vi "ble_read_write_characteristics.vi"() -> ()   [LabVIEW 2013]
uses:
  type_def/connection_status_bundle.ctl
  type_def/address_type.ctl
  ble_functions/ble_write_by_service_characteristic_uint8array.vi
panel:
  out "Connected":bool
  out "Device Name":string
  in  "Address Type":T1=1 items=["Public", "Random"]
  out "Handle table":string[][](array[string])
  out "Connection Status":T2={"MAC Address"="", "cnx handle"=0, "cnx flags"=0, "Address Type"=125, "Connection Interval (ms)"=125, "Timeout(ms)"=125, "Latency"=0, "bonding handle"=0} {"Address Type" items=["Public", "Random"]}
  out "Scanning":bool
  in  "Continue":bool
  in  "MAC Address":string
  in  "COM Bluegiga in":refnum<visa-resource-name>="COM13"
  out "Devices":string[][](array[string])
  out "BLED112 Dongle Info":string
  # "This VI an example of scanning for BLE devices using the \nBLED112 Bluetooth Smart Dongle by Bluegiga\nhttps://www.bluegiga.com/en-US/products/bled112-bluetooth-smart-dongle/\n\nand\nBLE (Bluetooth Low Energy) toolkit for LabVIEW\nww.\n\nInstructions:\nBefore running the VI\n1. Select the COM port for the BLED112 USB receiver\n(You can verify this in the Device Manager)\n\n2. Run the VI\n\n3. The VI will reset the dongle and scan for available BLE devices\n \n4. Introduce the MAC Address and Address Type of the device you want to connect and click in the CONTINUE button to connect with it\n\n5. The VI will read the Characteristic 0x2A00 of the Service 0x1800 which contains \nthe Device Name\n\nhttps://www.bluetooth.com/specifications/gatt/viewer?attributeXmlFile=org.bluetooth.service.generic_access.xml&u=org.bluetooth.service.generic_access.xml"
  # "SCAN"
  # "RSSI (power)"
  # "Advertising Package Type"
  # "MAC Address"
  # "Address Type"
  # "Friendly name"
  # "DEVICES FOUND"
  # "Introduce the MAC Address and Address Type of the device you want to connect and click in the CONTINUE button"
  # "CONNECT"
  # "READING DEVICE NAME"
  # "Service 0x1800\nCharacteristic 0x2A00\nDevice Name"
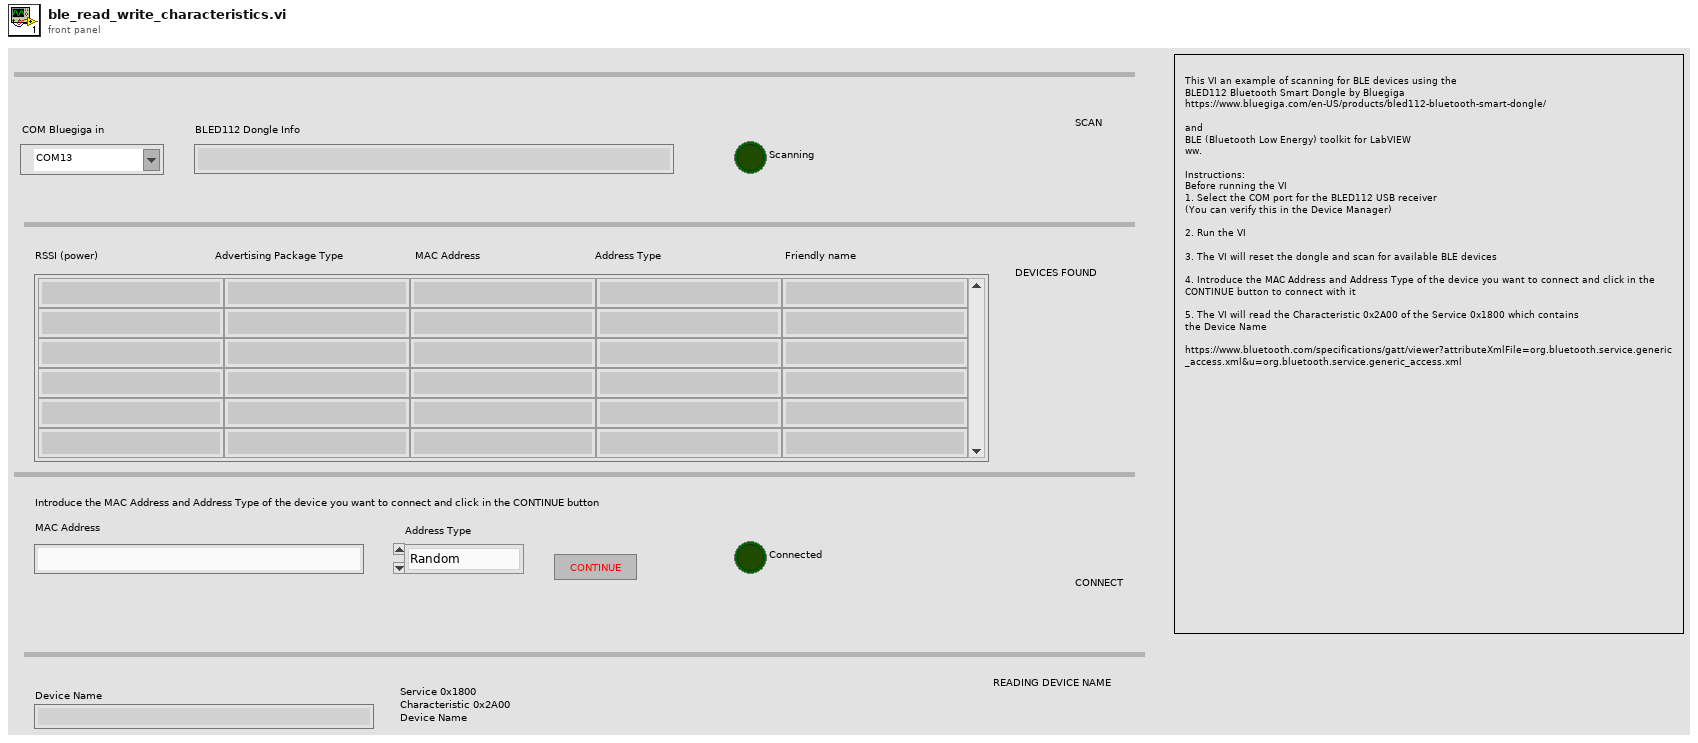
[diagram p1: front panel]
types:
  T1 = typedef "address_type.ctl" = u8
  T2 = typedef "connection_status_bundle.ctl" = cluster{"MAC Address":string, "cnx handle":u8, "cnx flags":u8, "Address Type":T1, "Connection Interval (ms)":u16, "Timeout(ms)":u16, "Latency":u16, "bonding handle":u8}
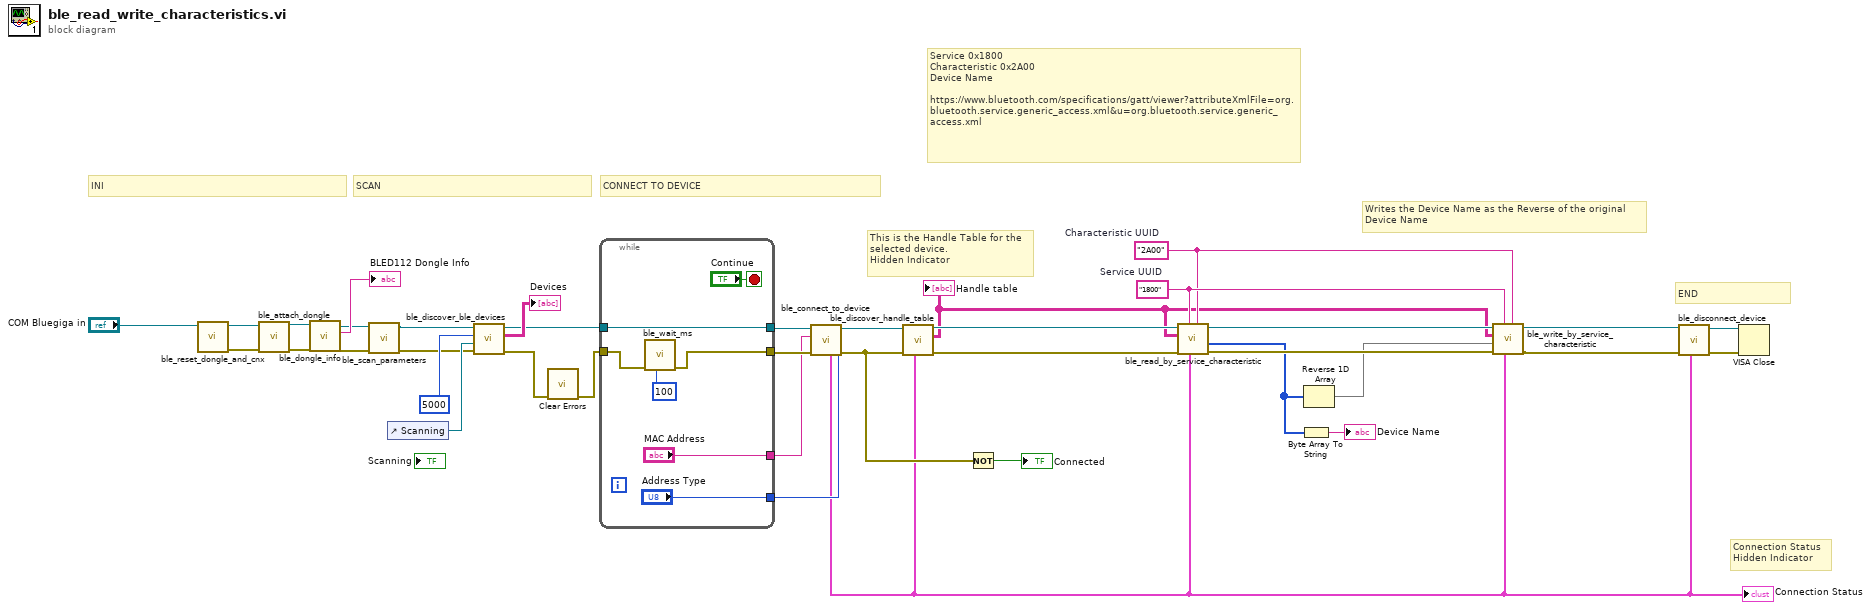
[diagram p0: block diagram]
diagram:
  w6 = "2A00"  # Characteristic UUID
  w7 = "1800"  # Service UUID
  # "Writes the Device Name as the Reverse of the original\nDevice Name"
  # "Connection Status\nHidden Indicator"
  # "Service 0x1800\nCharacteristic 0x2A00\nDevice Name\n\nhttps://www.bluetooth.com/specifications/gatt/viewer?attributeXmlFile=org.bluetooth.service.generic_access.xml&u=org.bluetooth.service.generic_access.xml"
  # "This is the Handle Table for the\nselected device. \nHidden Indicator"
  # "CONNECT TO DEVICE"
  # "SCAN"
  # "END"
  # "INI"
  n1 = call "ble_reset_dongle_and_cnx.vi"("COM Bluegiga in"="COM Bluegiga in") -> ("error out"=w22:errorcluster, "COM Bluegiga out"=w20:refnum<visa-resource-name>)  [unwired: 9 in]
  n2 = call "ble_attach_dongle.vi"("error in (no error)"=w22, "COM Bluegiga in"=w20) -> ("error out"=w24:errorcluster, "COM Bluegiga out"=w23:refnum<visa-resource-name>)  [unwired: 8 in]
  n3 = call "ble_dongle_info.vi"("error in (no error)"=w24, "COM Bluegiga in"=w23) -> ("error out"=w30:errorcluster, "info"=→"BLED112 Dongle Info":string, "COM Bluegiga out"=w31:refnum<visa-resource-name>)  [unwired: 7 in]
  n4 = call "ble_scan_parameters.vi"("error in (no error)"=w30, "COM Bluegiga in"=w31) -> ("error out"=w28:errorcluster, "COM Bluegiga out"=w29:refnum<visa-resource-name>)  [unwired: 7 in, 1 out]
  n5 = control-ref of="Scanning"() -> (w34:refnum<vi>)
  n6 = call "ble_discover_ble_devices.vi"("error in (no error)"=w28, "LED ref"=w34, "Scan Duration (10000ms)"=u32 5000, "COM Bluegiga in"=w29) -> ("error out"=w18:errorcluster, "Devices"=→"Devices":string[][], "COM Bluegiga out"=w35:refnum<visa-resource-name>)  [unwired: 5 in]
  n7 = call <vilib>:"Clear Errors.vi"("error in (no error)"=w18) -> ("error out"=w17:errorcluster)  [unwired: 6 in]
  n8 = while {
    tunnel: w17 -> [w44]
    tunnel: [w43] -> w33
    tunnel: w35 -> [w43]
    tunnel: [w42] -> w32
    tunnel: ["MAC Address"] -> w25
    tunnel: ["Address Type"] -> w16
    stop <- "Continue" stop-if-true
    n9 = call "ble_wait_ms.vi"("milliseconds to wait (100)"=u32 100, "error in (no error)"=w44) -> ("error out"=w42:errorcluster)  [unwired: 9 in]
  }
  n10 = call "ble_connect_to_device.vi"("Address Type"=w16, "error in (no error)"=w32, "MAC Address"=w25, "COM Bluegiga in"=w33) -> ("error out"=w11:errorcluster, "COM Bluegiga out"=w19:refnum<visa-resource-name>, "Connection Status"=w8:T2)  [unwired: 5 in]
  "Connection Status" <- w8
  n11 = call "ble_discover_handle_table.vi"("Connection Status"=w8, "error in (no error)"=w11, "COM Bluegiga in"=w19) -> ("error out"=w15:errorcluster, "Handle table"=w5:string[][], "COM Bluegiga out"=w14:refnum<visa-resource-name>)  [unwired: 6 in]
  "Handle table" <- w5
  n12 = Not(x=w11) -> (.not. x?=→"Connected":bool)
  n13 = call "ble_read_by_service_characteristic.vi"("Characteristic UUID"=w6, "Connection Status"=w8, "Service UUID"=w7, "error in (no error)"=w15, "Handle table"=w5, "COM Bluegiga in"=w14) -> ("error out"=w9:errorcluster, "attribute value"=w1:u8[], "COM Bluegiga out"=w10:refnum<visa-resource-name>)  [unwired: 2 in, 1 out]
  n14 = Byte Array To String(unsigned byte array=w1) -> (string=→"Device Name":string)
  n15 = Reverse 1D Array(array=w1) -> (reversed array=w4:u8[])
  n16 = call-poly "ble_write_by_service_characteristic.vi"("Characteristic UUID"=w6, "Connection Status"=w8, "Service UUID"=w7, "error in (no error)"=w9, "data"=w4, "Handle table"=w5, "COM Bluegiga in"=w10) -> ("error out"=w3:errorcluster, "COM Bluegiga out"=w2:refnum<visa-resource-name>)  [unwired: 3 in]
  n17 = call "ble_disconnect_device.vi"("Connection Status"=w8, "error in (no error)"=w3, "COM Bluegiga in"=w2) -> ("error out"=w26:errorcluster, "COM Bluegiga out"=w27:refnum<visa-resource-name>)  [unwired: 7 in]
  n18 = VISA Close(VISA resource name=w27, error in (no error)=w26) -> ()  [unwired: 1 out]
